vi "UnHookWindowProc.vi"(4 "error in (no error)":errorcluster, 6 "hWnd":T1, 7 "siwutil32":T2) -> (0 "error out":errorcluster)   [LabVIEW 2011]
uses:
  siwutil32.ctl
  WinUSER/Windows/hWnd.ctl
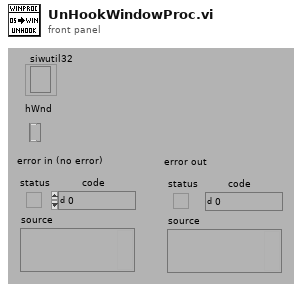
[diagram p1: front panel]
types:
  T1 = typedef "hWnd.ctl" = refnum<k1>
  T2 = typedef "siwutil32.ctl" = refnum<k7>
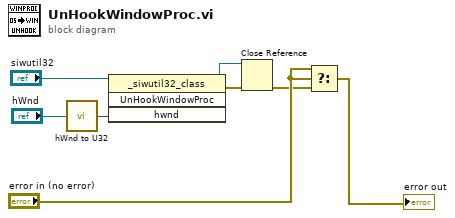
[diagram p0: block diagram]
diagram:
  n1 = call "hWnd to U32.vi"("hWnd"="hWnd") -> ("hWnd"=w4:u32)  [unwired: 4 out]
  n2 = invoke class="_siwutil32_class" method="UnHookWindowProc"(reference="siwutil32", "hwnd"=w4) -> (reference out=w8:T2, error out=w7:errorcluster)  [unwired: 2 in, 2 out]
  n3 = Close Reference(reference=w8, error in (no error)=w7) -> (error out=w2:errorcluster)
  n4 = Select(t="error in (no error)", s="error in (no error)", f=w2) -> (s? t:f=→"error out":errorcluster)
